vi "Get Event Reference.vi"(4 "error in (no error)":errorcluster) -> (0 "error out":errorcluster, 3 "Set TC Parameters":refnum<user-event>)   [LabVIEW 2015, in "Set TC Parameters.lvlib"]
uses:
  Set TC Parameters.lvlib
  _typedefs/Event Data.ctl
  _libraries/Startup Processes/_typedefs/TC Setup Parameters.ctl
  _libraries/Startup Processes/Startup Processes.lvlib
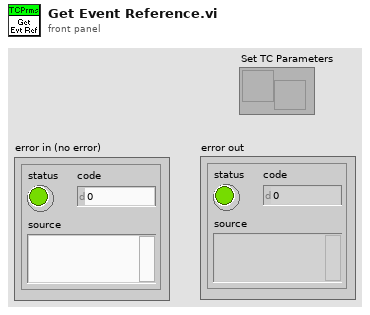
[diagram p1: front panel]
types:
  T1 = typedef "Set TC Parameters.lvlib/Event Data.ctl" = cluster{"Plugin Name":string, "TC Parameters":T2, "Response Notifier":string}
  T2 = typedef "Startup Processes.lvlib/TC Setup Parameters.ctl" = cluster{"Error High Level":dbl, "Warning High Level":dbl, "Warning Low Level":dbl, "Error Low Level":dbl, "Sample Interval":dbl[unit]}
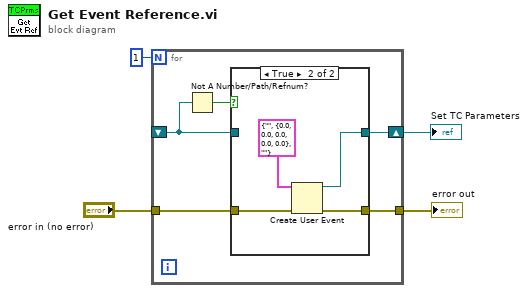
[diagram p0: block diagram]
diagram:
  n1 = for {
    N: 1 -> [_]
    shift-right: [w6] -> w4
    shift-left: _ -> [w8]
    tunnel: "error in (no error)" -> [w7]
    tunnel: [w5] -> w1
    n2 = Not A Number/Path/Refnum?(number/path/refnum=w8) -> (NaN/Path/Refnum?=w9:bool)
    n3 = case shown="True" w9 {
      tunnel: w8 -> [w11 _]
      tunnel: w7 -> [w10 w15]
      tunnel: [w11 w14] -> w6
      tunnel: [w10 w13] -> w5
      frame False {
      }
      frame True {
        n4 = Create User Event(user event datatype=T1 {"Plugin Name"="", "TC Parameters"={"Error High Level"=0.0, "Warning High Level"=0.0, "Warning Low Level"=0.0, "Error Low Level"=0.0, "Sample Interval"=0.0}, "Response Notifier"=""} ("data"), error in=w15) -> (user event=w14:refnum<user-event>, error out=w13:errorcluster)
      }
    }
  }
  "error out" <- w1
  "Set TC Parameters" <- w4
